vi "synnax writer open Single.vi"(4 "start (now)":timestamp, 5 "err_on_unauthorized (F)":bool, 6 "enable_auto_commit (F)":bool, 7 "auto_index (F)":bool, 8 "error in":errorcluster, 9 "authorities (255 for all channels)":u8, 10 "channel in":u32, 11 "Synnax Client in":refnum<class "Synnax Client.lvclass">) -> (0 "error out":errorcluster, 2 "channel out":u32, 3 "writer out":refnum<class "Synnax Writer.lvclass">)   [LabVIEW 2026, in "synnax_clib.lvlib" / "Synnax Writer.lvclass"]
doc: "SYNNAX_EXPORT int32_t synnax_writer_open(\n SynnaxClient client,\n int64_t start,\n const uint32_t *channels,\n uint64_t channel_count,\n int32_t mode,\n int32_t enable_auto_commit,\n SynnaxWriter *out_writer,\n SynnaxError err\n);"
uses:
  Synnax Writer.lvclass
  Client/Synnax Client.lvclass
  Client/Synnax Client.lvclass/Synnax Client.ctl
  Synnax Writer.lvclass/Synnax Writer.ctl
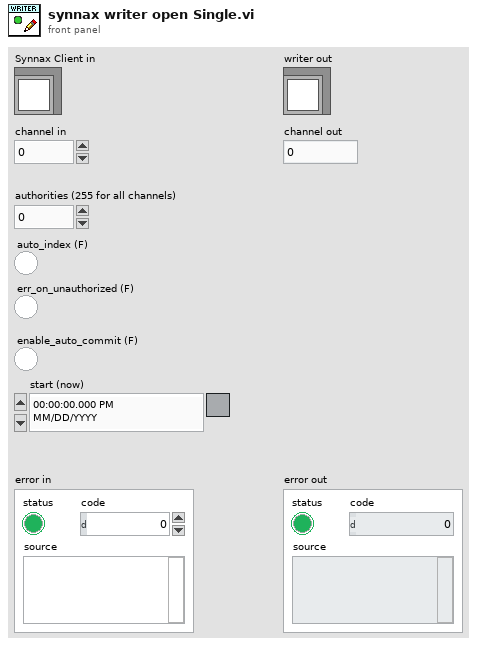
[diagram p1: front panel]
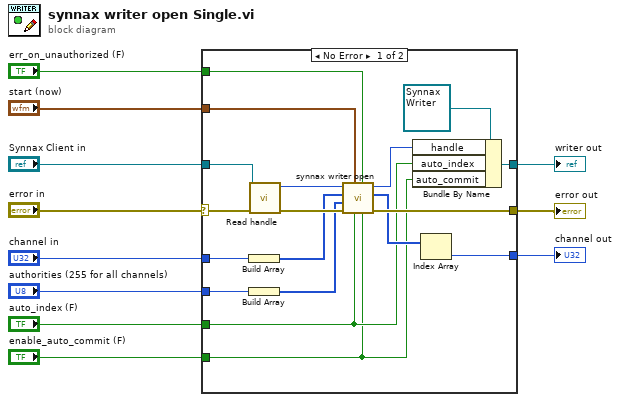
[diagram p0: block diagram]
diagram:
  n1 = case shown="No Error" "error in" {
    selector: "error in" -> [w14 w30]
    tunnel: "channel in" -> [w29 _]
    tunnel: "Synnax Client in" -> [w28 _]
    tunnel: "start (now)" -> [w26 _]
    tunnel: "authorities (255 for all channels)" -> [w24 _]
    tunnel: [w22 w30] -> w7
    tunnel: "err_on_unauthorized (F)" -> [w21 _]
    tunnel: "enable_auto_commit (F)" -> [w12 _]
    tunnel: "auto_index (F)" -> [w13 _]
    tunnel: [w20 _] -> w3
    tunnel: [w15 _] -> w2
    frame No Error {
      n2 = Build Array(w29) -> (w25:u32[])
      n3 = Build Array(w24) -> (w23:u8[])
      n4 = call "Read handle.vi"("error in (no error)"=w14, "Synnax Client in"=w28) -> ("error out"=w27:errorcluster, "handle"=w18:u64)  [unwired: 7 in, 1 out]
      n5 = call "synnax writer open.vi"("enable_auto_commit (F)"=w12, "err_on_unauthorized (F)"=w21, "auto_index (F)"=w13, "start (now)"=w26, "error in"=w27, "authorities (255 for all channels)"=w23, "channels"=w25, "sy client handle"=w18) -> ("error out"=w22:errorcluster, "channels out"=w19:u32[], "sy writer handle"=w16:u64)  [unwired: 1 in]
      n6 = Bundle By Name(cluster=refnum<class "Synnax Writer.lvclass"> refnum, "handle"=w16, "auto_index"=w13, "auto_commit"=w12) -> (w15:refnum<class "Synnax Writer.lvclass">)
      n7 = Index Array(array=w19) -> (element=w20:u32)  [unwired: 1 in]
    }
    frame Error {
    }
  }
  "error out" <- w7
  "channel out" <- w3
  "writer out" <- w2
